vi "Set Target Destination Directory.vi"(8 "error in (no error)":errorcluster, 10 "Target Destination Directory":path, 11 "BuildSpec in":refnum<vi>) -> (0 "error out":errorcluster, 3 "BuildSpec out":refnum<vi>)   [LabVIEW 2019, in "Project Sync Tools.lvclass"]
uses:
  Project Sync Tools.lvclass
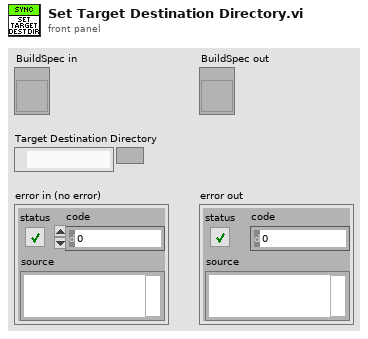
[diagram p1: front panel]
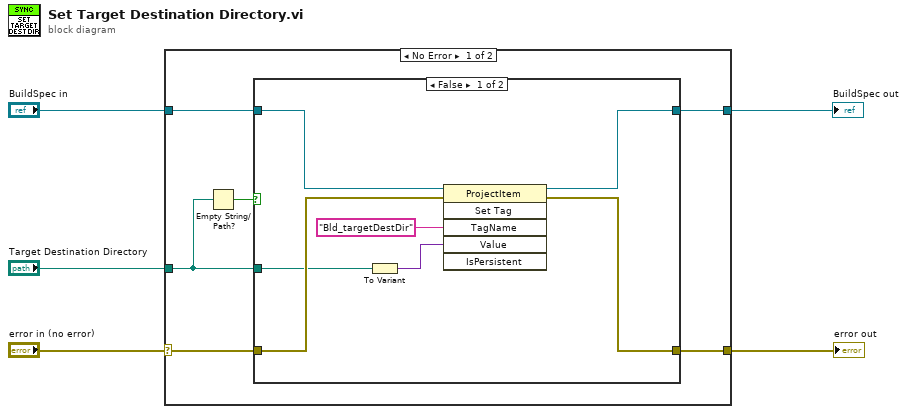
[diagram p0: block diagram]
diagram:
  n1 = case shown="No Error" "error in (no error)" {
    selector: "error in (no error)" -> [w8 w21]
    tunnel: [w11 w21] -> w5
    tunnel: "BuildSpec in" -> [w10 w22]
    tunnel: "Target Destination Directory" -> [w7 _]
    tunnel: [w9 w22] -> w2
    frame No Error {
      n2 = Empty String/Path?(string/path=w7) -> (empty?=w6:bool)
      n3 = case shown="False" w6 {
        tunnel: [w18 w19] -> w11
        tunnel: w10 -> [w17 w20]
        tunnel: [w14 w20] -> w9
        tunnel: w8 -> [w13 w19]
        tunnel: w7 -> [w12 _]
        frame False {
          n4 = To Variant(anything=w12) -> (Variant=w15:variant)
          n5 = invoke class="ProjectItem" method="Set Tag"(reference=w17, error in=w13, "TagName"="Bld_targetDestDir" ("Tag Name"), "Value"=w15) -> (reference out=w14:refnum<vi>, error out=w18:errorcluster)  [unwired: 2 in, 4 out]
        }
        frame True {
        }
      }
    }
    frame Error {
    }
  }
  "error out" <- w5
  "BuildSpec out" <- w2
